vi "Peregrine_read_motor_parameters.vi"(0 "Handle in":refnum<visa-resource-name>, 2 "Address":u8, 7 "Select parameter":T1(ring), 11 "error":errorcluster) -> (4 "Handle out":refnum<visa-resource-name>, 6 "Key response":u32, 8 "Raw value response":i32, 10 "Decoded value response":dbl, 15 "error out":errorcluster)   [LabVIEW 2019]
panel:
  # "Inputs"
  # "Response message"
  # "Output"
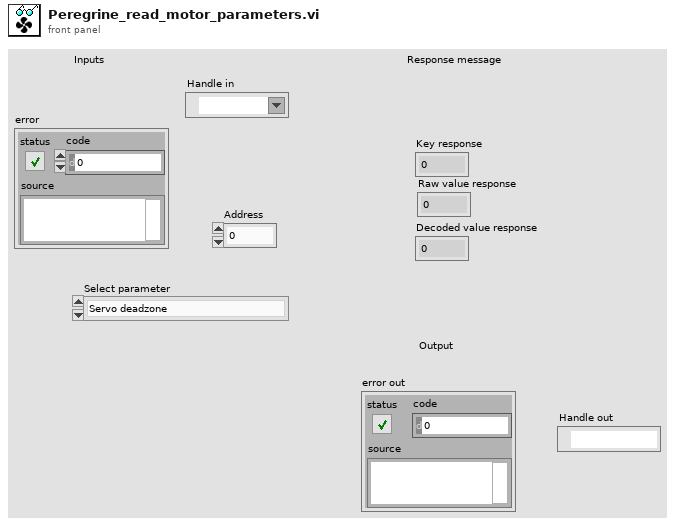
[diagram p1: front panel]
types:
  T1 = enum16{"Servo deadzone", "Position target gain", "Position target P", "Position target D", "V target P", "V target D", "Frequency slew", "Motor direction", "Error gain", "LQR K0", "LQR K1", "LQR B1", "Encoder DIV", "FDIR steprate"}
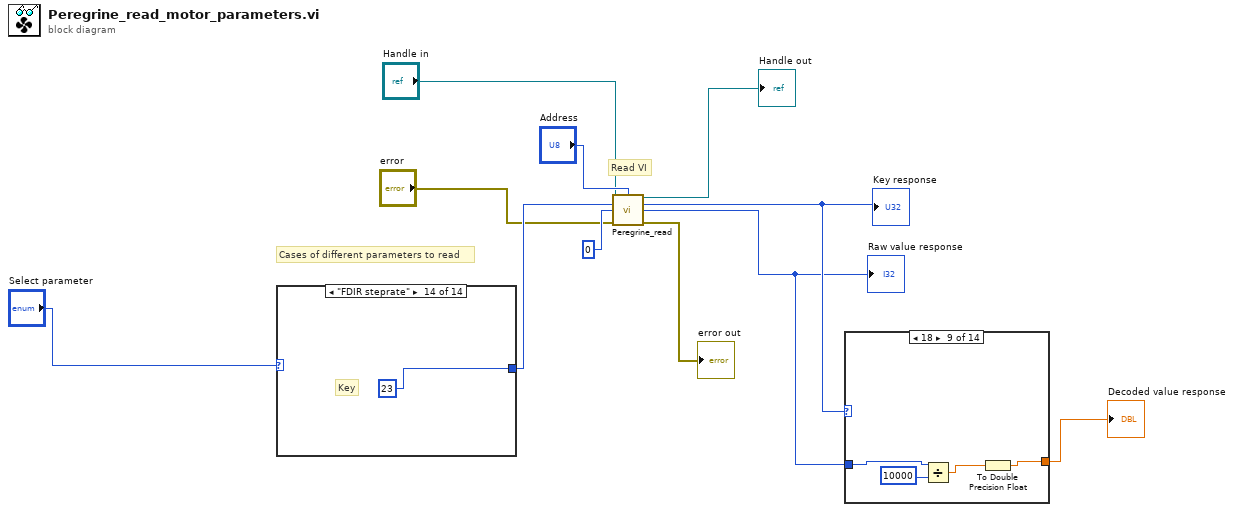
[diagram p0: block diagram]
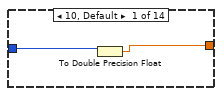
[diagram p2: hidden frame]
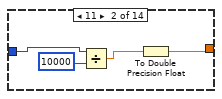
[diagram p3: hidden frame]
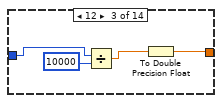
[diagram p4: hidden frame]
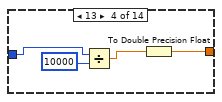
[diagram p5: hidden frame]
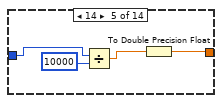
[diagram p6: hidden frame]
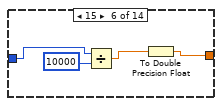
[diagram p7: hidden frame]
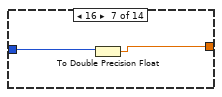
[diagram p8: hidden frame]
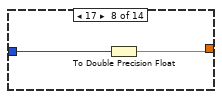
[diagram p9: hidden frame]
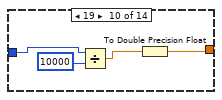
[diagram p10: hidden frame]
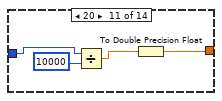
[diagram p11: hidden frame]
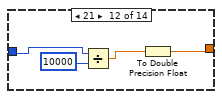
[diagram p12: hidden frame]
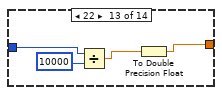
[diagram p13: hidden frame]
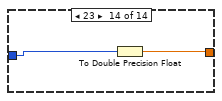
[diagram p14: hidden frame]
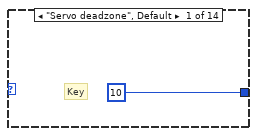
[diagram p15: hidden frame]
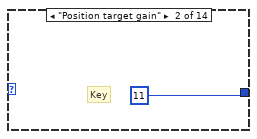
[diagram p16: hidden frame]
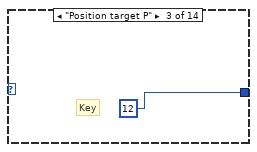
[diagram p17: hidden frame]
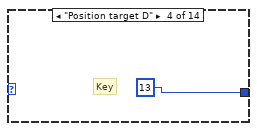
[diagram p18: hidden frame]
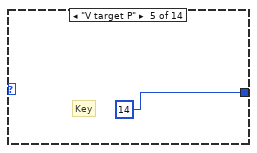
[diagram p19: hidden frame]
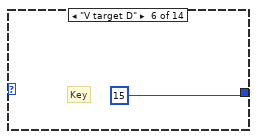
[diagram p20: hidden frame]
diagram:
  # "Cases of different parameters to read"
  # "Read VI"
  n1 = case shown="\"FDIR steprate\"" "Select parameter" {
    tunnel: [u32 10 u32 11 u32 12 u32 13 u32 14 u32 15 u32 16 u32 17 u32 18 u32 19 u32 20 u32 21 u32 22 u32 23] -> w8
    frame "Servo deadzone", Default {
      # "Key"
    }
    frame "Position target gain" {
      # "Key"
    }
    frame "Position target P" {
      # "Key"
    }
    frame "Position target D" {
      # "Key"
    }
    frame "V target P" {
      # "Key"
    }
    frame "V target D" {
      # "Key"
    }
    frame "Frequency slew" {
      # "Key"
    }
    frame "Motor direction" {
      # "Key"
    }
    frame "Error gain" {
      # "Key"
    }
    frame "LQR K0" {
      # "Key"
    }
    frame "LQR K1" {
      # "Key"
    }
    frame "LQR B1" {
      # "Key"
    }
    frame "Encoder DIV" {
      # "Key"
    }
    frame "FDIR steprate" {
      # "Key"
    }
  }
  n2 = call "Peregrine_read.vi"("Handle in"="Handle in", "Address"="Address", "Key"=w8, "Value"=0, "error"="error") -> ("Handle out"=→"Handle out":refnum<visa-resource-name>, "Key response"=w7:u32, "Value response"=w6:i32, "error out"=→"error out":errorcluster)  [unwired: 7 in]
  "Key response" <- w7
  "Raw value response" <- w6
  n3 = case shown="18" w7 {
    tunnel: w6 -> [w27 w29 w33 w37 w41 w45 w49 w51 w53 w57 w61 w64 w70 w73]
    tunnel: [w26 w28 w32 w36 w40 w44 w48 w50 w52 w56 w60 w65 w68 w72] -> w5
    frame 10, Default {
      n4 = To Double Precision Float(number=w27) -> (double precision float=w26:dbl)
    }
    frame 11 {
      n5 = Divide(x=w29, y=10000) -> (x/y=w30:dbl)
      n6 = To Double Precision Float(number=w30) -> (double precision float=w28:dbl)
    }
    frame 12 {
      n7 = Divide(x=w33, y=10000) -> (x/y=w34:dbl)
      n8 = To Double Precision Float(number=w34) -> (double precision float=w32:dbl)
    }
    frame 13 {
      n9 = Divide(x=w37, y=10000) -> (x/y=w38:dbl)
      n10 = To Double Precision Float(number=w38) -> (double precision float=w36:dbl)
    }
    frame 14 {
      n11 = Divide(x=w41, y=10000) -> (x/y=w42:dbl)
      n12 = To Double Precision Float(number=w42) -> (double precision float=w40:dbl)
    }
    frame 15 {
      n13 = Divide(x=w45, y=10000) -> (x/y=w46:dbl)
      n14 = To Double Precision Float(number=w46) -> (double precision float=w44:dbl)
    }
    frame 16 {
      n15 = To Double Precision Float(number=w49) -> (double precision float=w48:dbl)
    }
    frame 17 {
      n16 = To Double Precision Float(number=w51) -> (double precision float=w50:dbl)
    }
    frame 18 {
      n17 = Divide(x=w53, y=10000) -> (x/y=w54:dbl)
      n18 = To Double Precision Float(number=w54) -> (double precision float=w52:dbl)
    }
    frame 19 {
      n19 = Divide(x=w57, y=10000) -> (x/y=w58:dbl)
      n20 = To Double Precision Float(number=w58) -> (double precision float=w56:dbl)
    }
    frame 20 {
      n21 = Divide(x=w61, y=10000) -> (x/y=w62:dbl)
      n22 = To Double Precision Float(number=w62) -> (double precision float=w60:dbl)
    }
    frame 21 {
      n23 = Divide(x=w64, y=10000) -> (x/y=w66:dbl)
      n24 = To Double Precision Float(number=w66) -> (double precision float=w65:dbl)
    }
    frame 22 {
      n25 = Divide(x=w70, y=10000) -> (x/y=w69:dbl)
      n26 = To Double Precision Float(number=w69) -> (double precision float=w68:dbl)
    }
    frame 23 {
      n27 = To Double Precision Float(number=w73) -> (double precision float=w72:dbl)
    }
  }
  "Decoded value response" <- w5
